vi "质控启动流程对话框.vi"() -> (0 "确定启动":bool, 1 "启动模块":T1, 2 "直接启动":bool, 3 "常规启动":bool)   [LabVIEW 2016, in "质控单元.lvlib"]
uses:
  <vilib>/Utility/miscctls.llb/LVPointTypeDef.ctl
panel:
  in  "直接启动":bool
  in  "取消":bool
  in  "常规启动":bool
  # "请选择启动模式"
  # "常规启动：先启动采配水，再进行加标回收"
  # "直接启动：不启动采配水，直接加标回收"
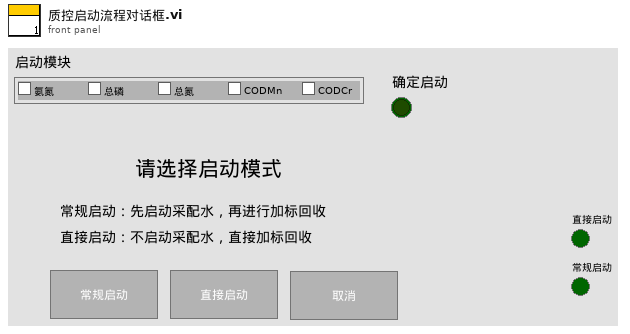
[diagram p1: front panel]
types:
  T1 = cluster{"氨氮":bool, "总磷":bool, "总氮":bool, "CODMn":bool, "CODCr":bool}
  T2 = typedef "LVPointTypeDef.ctl" = cluster{"Horizontal":i16, "Vertical":i16}
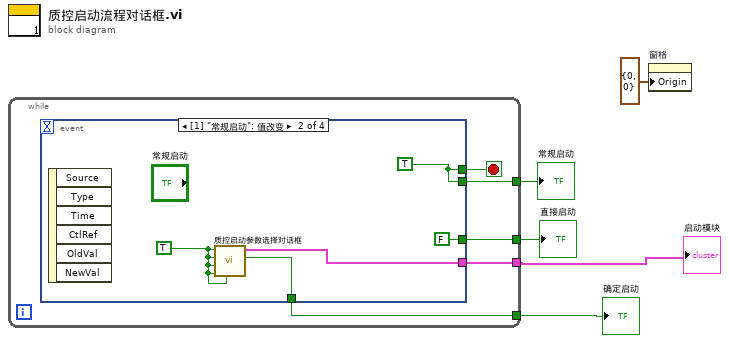
[diagram p0: block diagram]
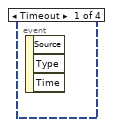
[diagram p2: hidden frame]
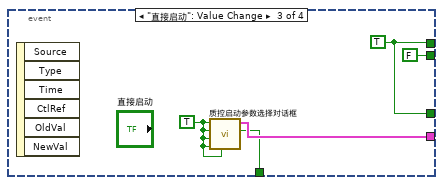
[diagram p3: hidden frame]
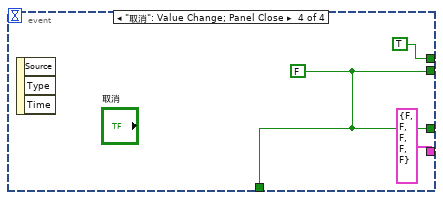
[diagram p4: hidden frame]
diagram:
  n1 = while {
    tunnel: [w9] -> w5
    tunnel: [w8] -> w4
    tunnel: [w7] -> w2
    tunnel: [w6] -> w3
    stop <- w10 stop-if-true
    n2 = event shown="[1] \"常规启动\": 值改变" {
      selector: _ -> [_ _ _ _]
      dyn-events: _ -> [_ _ _ _]
      timeout: _ -> [_ _ _ _]
      tunnel: [_ w15 w20 TRUE ("确定")] -> w10
      tunnel: [_ w15 FALSE ("确定") w22] -> w9
      tunnel: [_ FALSE ("确定") w20 w22] -> w8
      tunnel: [_ w13 w18 T1 {"氨氮"=FALSE, "总磷"=FALSE, "总氮"=FALSE, "CODMn"=FALSE, "CODCr"=FALSE} ("启动模块")] -> w7
      tunnel: [_ w12 w17 w22] -> w6
      event Timeout {
        n3 = event-data() -> ()  [unwired: 1 in, 3 out]
      }
      event "常规启动": Value Change {
        w11 = TRUE ("氨氮")
        w15 = TRUE ("确定")
        n4 = event-data() -> ()  [unwired: 1 in, 6 out]
        n5 = call "质控启动参数选择对话框.vi"("CODCr"=w11, "CODMn"=w11, "总氮"=w11, "总磷"=w11, "氨氮"=w11) -> ("确定启动"=w12:bool, "启动模块"=w13:T1)  [unwired: 4 in, 1 out]
      }
      event "直接启动": Value Change {
        w16 = TRUE ("氨氮")
        w20 = TRUE ("确定")
        n6 = event-data() -> ()  [unwired: 1 in, 6 out]
        n7 = call "质控启动参数选择对话框.vi"("CODCr"=w16, "CODMn"=w16, "总氮"=w16, "总磷"=w16, "氨氮"=w16) -> ("确定启动"=w17:bool, "启动模块"=w18:T1)  [unwired: 4 in, 1 out]
      }
      event "取消": Value Change; Panel Close {
        w22 = FALSE ("确定")
        n8 = event-data() -> ()  [unwired: 1 in, 3 out]
      }
    }
  }
  "常规启动" <- w5
  "直接启动" <- w4
  "确定启动" <- w3
  "启动模块" <- w2
  n9 = property on="窗格" class="Pane"("Origin"=T2 {"Horizontal"=0, "Vertical"=0} ("原点")) -> ()  [unwired: 2 in, 2 out]
